vi "ECC_v1.vi"() -> ()   [LabVIEW 2013]
uses:
  state_machine.ctl
  <vilib>/DAQmx/write.llb/DAQmx Write (Analog Wfm 1Chan NSamp).vi
  <vilib>/DAQmx/create/channels.llb/DAQmx Create Channel (AO-Voltage-Basic).vi
  <vilib>/DAQmx/configure/timing.llb/DAQmx Timing (Use Waveform).vi
  <vilib>/DAQmx/miscellaneous.llb/DAQmx Fill In Error Info.vi
panel:
  in  "R&S/5181":bool=TRUE
  out "on_bad_status":bool
  out "off_bad_status":bool
  out "Pause, s":i32
  out "APS_off_status":bool=TRUE
  out "R&S_off_status":bool=TRUE
  out "Countdown":u32
  in  "Rep_delay":u32
  in  "Finite/Continuous":bool
  in  "ResumeSweep":bool
  in  "PauseSweep":bool
  in  "RF_off_rep":bool
  in  "RF_off_set":bool
  in  "RF_off_cycle":bool
  in  "APS_off_rep":bool=TRUE
  in  "APS_off_set":bool
  in  "APS_off_cycle":bool
  in  "AbortSweep":bool
  in  "Check APS":bool
  in  "ON/OFF_APS":bool
  in  "Check R&S":bool
  in  "ON/OFF_RF":bool
  in  "Use_APS":bool=TRUE
  out "DAC_status":bool
  out "RF_status":bool
  out "i_Current_repetition":i32
  out "N_Cycles_Created":i32
  out "i_Current_cycle":i32
  in  "M_repetitions":i32 min=0
  in  "Set_of_Cycles":T1(array[cluster])=[{"On/Off"=TRUE, "f0, MHz"=32.5, "fm, kHz"=100, "A, mV"=20, "Waveform"=enum."triangle", "N_steps"=500, "T_sweep, s"=0.1, "N_sweeps"=5, "End_Wait, s"=0}] {"End_Wait, s" step=1; "N_sweeps" min=0 step=1; "T_sweep, s" min=0.0 step=0.001 format="%#_6f"; "N_steps" min=0 step=1; "fm, kHz" step=1; "f0, MHz" min=0.0 step=0.001 format="%#_6f"}
  out "APS_status":bool
  in  "APS address":refnum<visa-resource-name>="COM3"
  in  "Init Devices":bool
  in  "Do Sweep":bool
  in  "Exit":bool
  in  "DAC channel":tag="Dev1/ao0"
  in  "RF address":string(combo)="29"
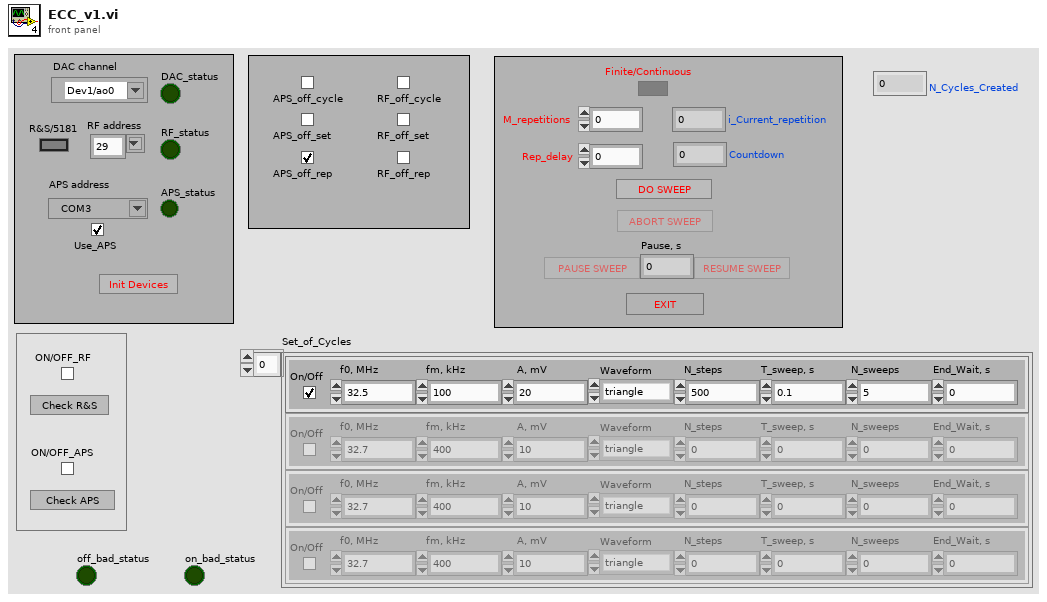
[diagram p1: front panel]
types:
  T1 = cluster{"On/Off":bool, "f0, MHz":dbl, "fm, kHz":i32, "A, mV":i32, "Waveform":enum16{"triangle", "saw_direct", "saw_invert", "sine"}, "N_steps":i32, "T_sweep, s":dbl, "N_sweeps":i32, "End_Wait, s":u32}[]
  T2 = typedef "state_machine.ctl" = enum16{"idle", "init_daq", "init_rf", "init_ps", "cycle_start", "get_wf", "rf_on", "rf_off", "rf_set", "ps_on", "ps_off", "daq_start", "daq_stop", "daq_wait", "daq_dt", "daq_v", "delay", "cycle_reset", "exit", "repetition_reset"}
  T3 = enum8{"Enabled", "Disabled", "Disabled and Grayed Out"}
  T4 = cluster{"On/Off":bool, "f0, MHz":dbl, "fm, kHz":i32, "A, mV":i32, "Waveform":enum16{"triangle", "saw_direct", "saw_invert", "sine"}, "N_steps":i32, "T_sweep, s":dbl, "N_sweeps":i32, "End_Wait, s":u32}
  T5 = enum16{"triangle", "saw_direct", "saw_invert", "sine"}
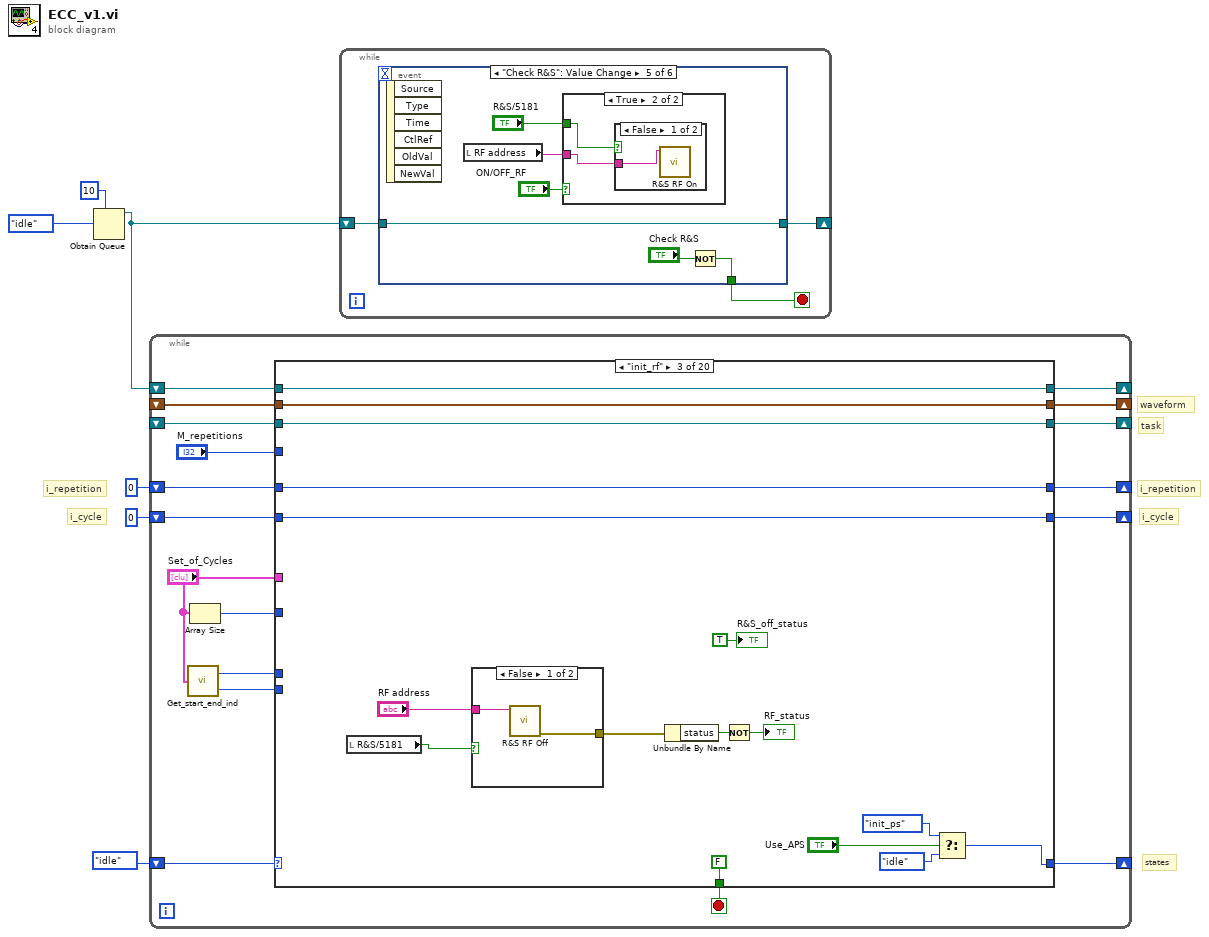
[diagram p0: block diagram]
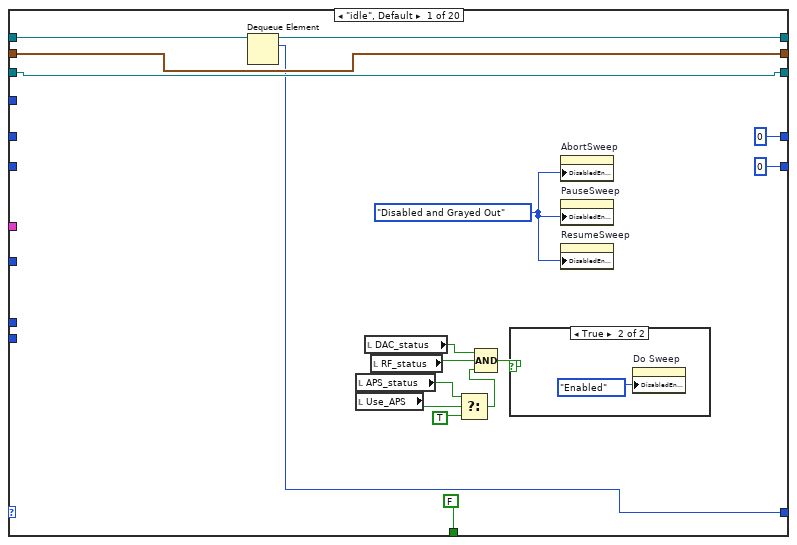
[diagram p2: hidden frame]
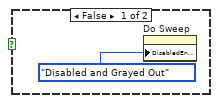
[diagram p3: hidden frame]
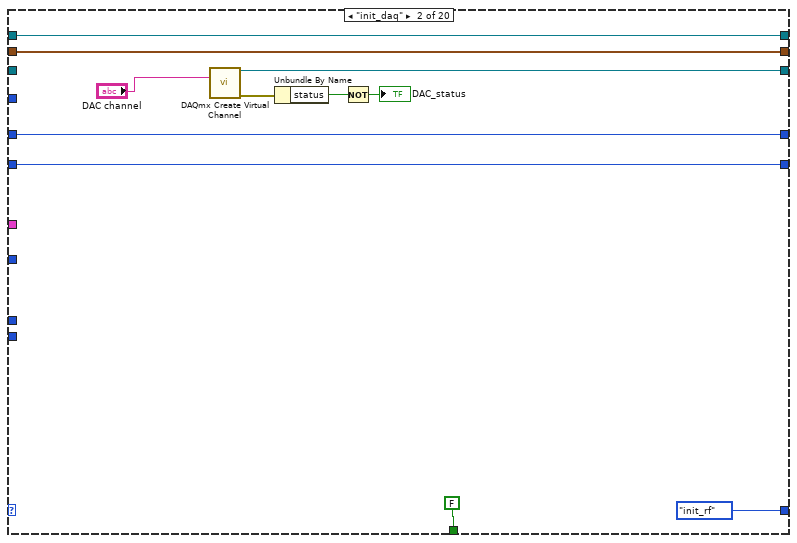
[diagram p4: hidden frame]
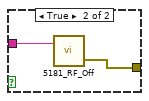
[diagram p5: hidden frame]
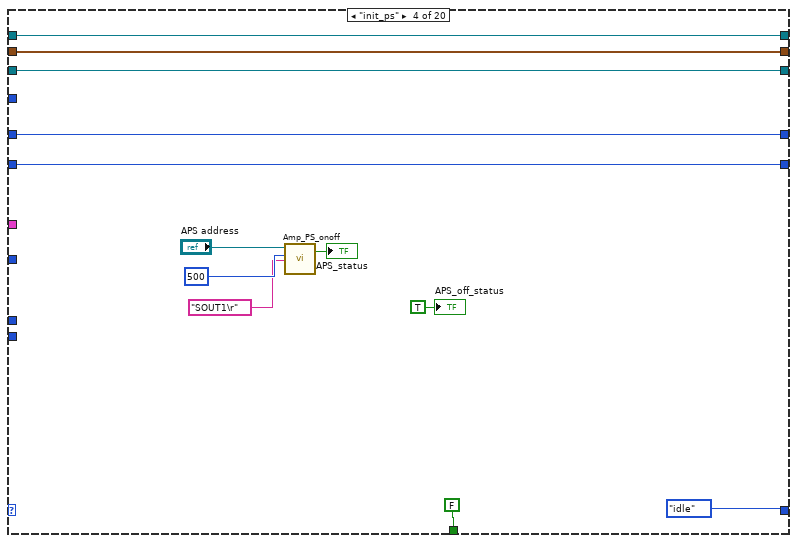
[diagram p6: hidden frame]
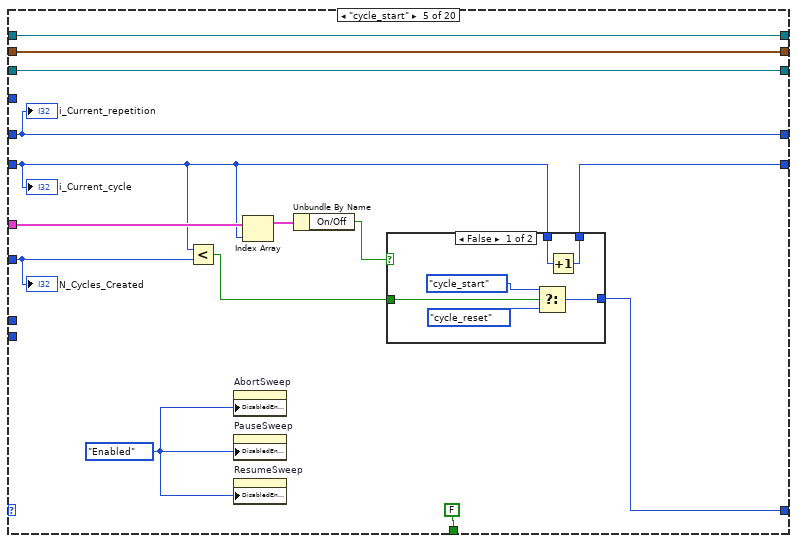
[diagram p7: hidden frame]
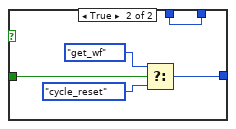
[diagram p8: hidden frame]
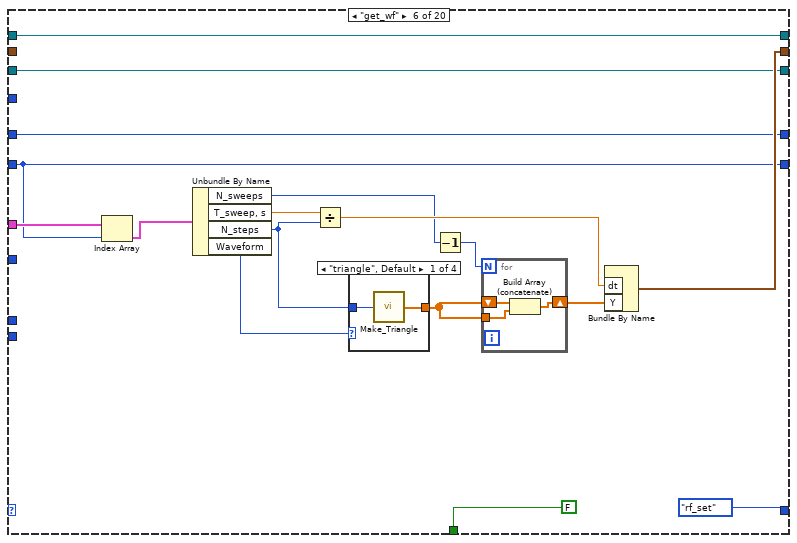
[diagram p9: hidden frame]
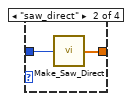
[diagram p10: hidden frame]
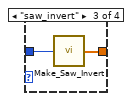
[diagram p11: hidden frame]
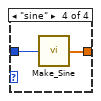
[diagram p12: hidden frame]
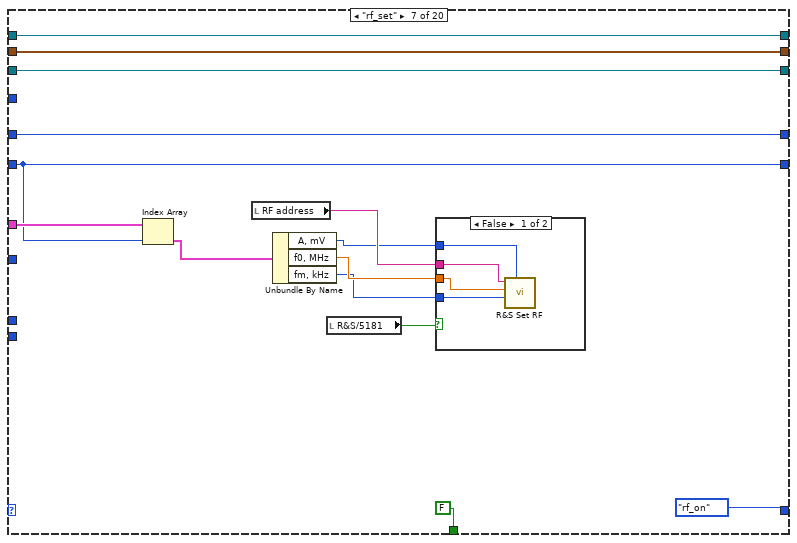
[diagram p13: hidden frame]
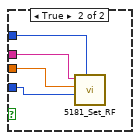
[diagram p14: hidden frame]
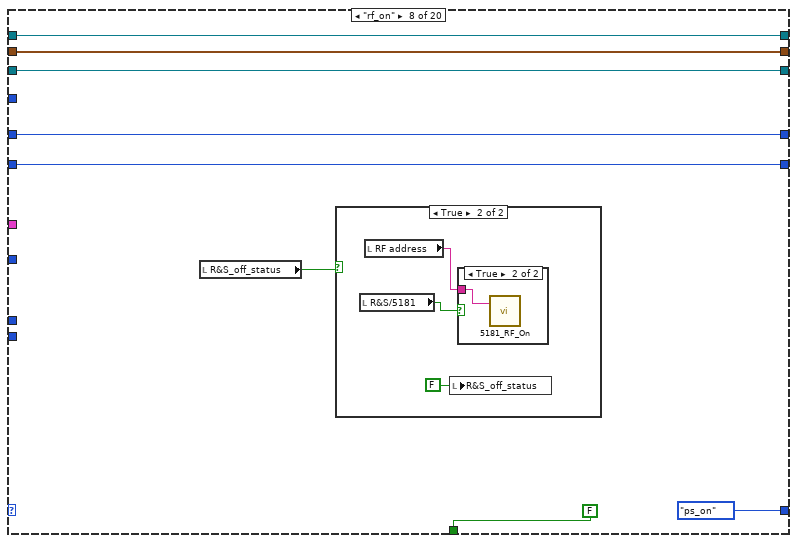
[diagram p15: hidden frame]
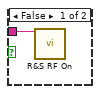
[diagram p17: hidden frame]
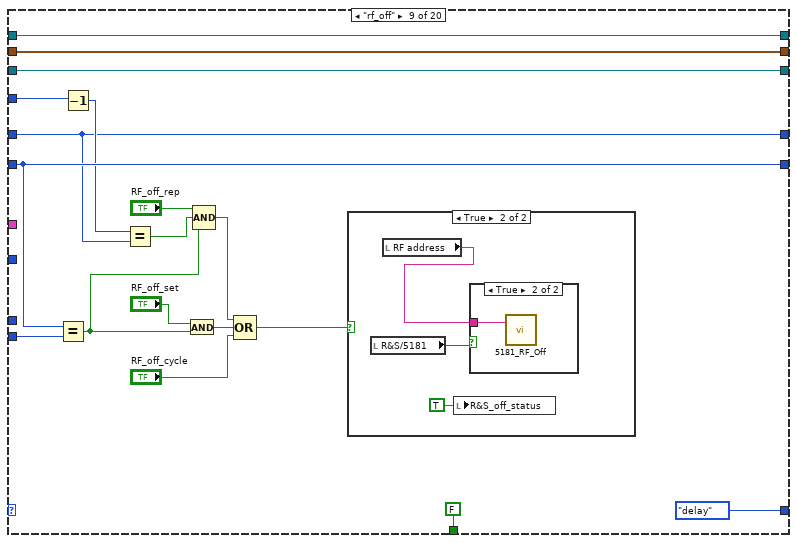
[diagram p18: hidden frame]
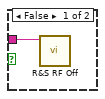
[diagram p20: hidden frame]
diagram:
  # "i_repetition"
  # "i_cycle"
  # "i_repetition"
  # "i_cycle"
  # "states"
  # "waveform"
  # "task"
  n1 = Obtain Queue(max queue size (-1, unlimited)=10, element data type=state_machine."idle") -> (queue out=w4:refnum<queue>)  [unwired: 3 in, 2 out]
  n2 = while {
    shift-right: [w19] -> _
    shift-left: state_machine."idle" -> [w24]
    shift-right: [w23] -> _
    shift-left: _ -> [w21]
    shift-right: [w22] -> _
    shift-left: _ -> [w20]
    shift-right: [w17] -> _
    shift-left: w4 -> [w18]
    shift-right: [w15] -> _
    shift-left: 0 -> [w14]
    shift-right: [w13] -> _
    shift-left: 0 -> [w12]
    stop <- w16 stop-if-true
    n3 = call "Get_start_end_ind.vi"("Set_of_Cycles"="Set_of_Cycles") -> ("start_ind"=w9:i32, "end_ind"=w8:i32)
    n4 = Array Size(array="Set_of_Cycles") -> (size(s)=w11:i32)
    n5 = case shown="\"init_rf\"" w24 {
      selector: w24 -> [_ _ _ _ _ _ _ _ _ _ _ _ _ _ _ _ _ _ w360 _]
      tunnel: [w40 w52 w69 w85 w89 w120 w149 w166 w189 w206 w223 w248 w256 w264 w273 w280 w292 w310 w357 w368] -> w23
      tunnel: "Set_of_Cycles" -> [_ _ _ _ w99 w127 w151 _ _ _ _ _ _ _ _ _ w289 _ _ _]
      tunnel: [w39 w51 w68 w84 w90 w121 w148 w167 w190 w205 w222 w247 w255 w263 w272 w281 w293 w309 w356 w369] -> w22
      tunnel: w21 -> [w40 _ w69 w85 w89 w120 w149 w166 w189 w206 w223 w249 w257 w265 w274 w282 w292 w310 w357 w368]
      tunnel: w20 -> [w39 w51 w68 w84 w90 _ w148 w167 w190 w205 w222 w247 w255 w263 w272 w281 w293 w309 w356 w369]
      tunnel: [w36 state_machine."init_rf" w59 state_machine."idle" w95 state_machine."rf_set" state_machine."rf_on" state_machine."ps_on" state_machine."delay" state_machine."daq_dt" state_machine."rf_off" state_machine."daq_wait" state_machine."ps_off" state_machine."daq_stop" state_machine."daq_v" state_machine."daq_start" state_machine."cycle_start" w308 w360 w364] -> w19
      tunnel: w18 -> [w38 w48 w66 w81 w88 w118 w146 w168 w191 w202 w219 w244 w252 w260 w268 w277 w294 w311 w359 w371]
      tunnel: [w37 w48 w66 w81 w88 w118 w146 w168 w191 w202 w219 w244 w252 w260 w268 w277 w294 w311 w359 w371] -> w17
      tunnel: [FALSE FALSE FALSE FALSE FALSE FALSE FALSE FALSE FALSE FALSE FALSE FALSE FALSE FALSE FALSE FALSE FALSE FALSE TRUE FALSE] -> w16
      tunnel: w11 -> [_ _ _ _ w91 _ _ _ _ _ _ _ _ _ _ _ _ _ _ _]
      tunnel: [0 w47 w65 w80 w94 w111 w144 w162 w185 w200 w217 w243 w251 w259 w267 w276 w284 0 w355 w370] -> w15
      tunnel: w14 -> [_ w47 w65 w80 w92 w111 w144 w162 w185 w200 w217 w243 w251 w259 w267 w276 w283 _ w355 w370]
      tunnel: [0 w46 w64 w79 w87 w113 w145 w165 w177 w201 w212 w242 w250 w258 w266 w275 w291 w305 w354 0] -> w13
      tunnel: w12 -> [_ w46 w64 w79 w87 w113 w145 w165 w177 w201 w212 w242 w250 w258 w266 w275 w291 w306 w354 _]
      tunnel: "M_repetitions" -> [_ _ _ _ _ _ _ _ w182 _ w214 _ _ _ _ _ _ w313 _ _]
      tunnel: w9 -> [_ _ _ _ _ _ _ _ _ _ _ _ _ _ _ _ _ _ _ _]
      tunnel: w8 -> [_ _ _ _ _ _ _ _ w186 _ w218 _ _ _ _ _ _ _ _ _]
      frame "idle", Default {
        w25 = T3."Disabled and Grayed Out" ("Disabled")
        n6 = Dequeue Element(queue=w38) -> (queue out=w37:refnum<queue>, element=w36:T2)  [unwired: 2 in, 2 out]
        n7 = local read "APS_status"() -> (w28:bool)
        n8 = local read "Use_APS"() -> (w30:bool)
        n9 = local read "DAC_status"() -> (w32:bool)
        n10 = local read "RF_status"() -> (w31:bool)
        n11 = Select(t=w28, s=w30, f=TRUE) -> (s? t:f=w27:bool)
        n12 = Compound Arithmetic op=AND(w32, w31, w27) -> (w26:bool)
        n13 = case shown="True" w26 {
          frame False {
            n14 = property on="Do Sweep" class="Bool"("DisabledEnum"=T3."Disabled and Grayed Out" ("Disabled")) -> ()  [unwired: 2 in, 2 out]
          }
          frame True {
            n15 = property on="Do Sweep" class="Bool"("DisabledEnum"=T3."Enabled" ("Disabled")) -> ()  [unwired: 2 in, 2 out]
          }
        }
        n16 = property on="AbortSweep" class="Bool"("DisabledEnum"=w25) -> ()  [unwired: 2 in, 2 out]
        n17 = property on="PauseSweep" class="Bool"("DisabledEnum"=w25) -> ()  [unwired: 2 in, 2 out]
        n18 = property on="ResumeSweep" class="Bool"("DisabledEnum"=w25) -> ()  [unwired: 2 in, 2 out]
      }
      frame "init_daq" {
        n19 = call-poly <vilib>:"DAQmx Create Virtual Channel.vi"("physical channels"="DAC channel") -> ("task out"=w52:refnum<k21>, "error out"=w45:errorcluster)  [unwired: 13 in]
        n20 = Unbundle By Name(w45) -> ("status"=w44:bool)
        n21 = Not(x=w44) -> (.not. x?=→"DAC_status":bool)
      }
      frame "init_rf" {
        n22 = local read "R&S/5181"() -> (w54:bool)
        n23 = case shown="False" w54 {
          tunnel: "RF address" -> [w71 w73]
          tunnel: [w70 w72] -> w55
          frame False {
            n24 = call "R&S RF Off.vi"("address"=w71) -> ("error out"=w70:errorcluster)  [unwired: 5 in, 1 out]
          }
          frame True {
            n25 = call "5181_RF_Off.vi"("address"=w73) -> ("error out"=w72:errorcluster)  [unwired: 1 in, 1 out]
          }
        }
        n26 = Unbundle By Name(w55) -> ("status"=w62:bool)
        n27 = Not(x=w62) -> (.not. x?=→"RF_status":bool)
        n28 = Select(t=state_machine."init_ps", s="Use_APS", f=state_machine."idle") -> (s? t:f=w59:T2)
        "R&S_off_status" <- TRUE ("R&S_off_status")
      }
      frame "init_ps" {
        n29 = call "Amp_PS_onoff.vi"("On/Off Control"="SOUT1\r", "delay before read (ms)"=u32 500, "Amp PS address"="APS address") -> ("status"=→"APS_status":bool)  [unwired: 1 in, 1 out]
        "APS_off_status" <- TRUE ("APS_off_status")
      }
      frame "cycle_start" {
        w86 = T3."Enabled" ("Disabled")
        n30 = Less?(x=w92, y=w91) -> (x < y?=w96:bool)
        n31 = property on="AbortSweep" class="Bool"("DisabledEnum"=w86) -> ()  [unwired: 2 in, 2 out]
        n32 = property on="PauseSweep" class="Bool"("DisabledEnum"=w86) -> ()  [unwired: 2 in, 2 out]
        n33 = property on="ResumeSweep" class="Bool"("DisabledEnum"=w86) -> ()  [unwired: 2 in, 2 out]
        n34 = Index Array(array=w99, index=w92) -> (element=w98:T4)
        n35 = Unbundle By Name(w98) -> ("On/Off"=w97:bool)
        n36 = case shown="False" w97 {
          tunnel: w96 -> [w103 w109]
          tunnel: [w100 w108] -> w95
          tunnel: w92 -> [w105 w106]
          tunnel: [w104 w106] -> w94
          frame False {
            n37 = Select(t=state_machine."cycle_start", s=w103, f=state_machine."cycle_reset") -> (s? t:f=w100:T2)
            n38 = Increment(x=w105) -> (x+1=w104:i32)
          }
          frame True {
            n39 = Select(t=state_machine."get_wf", s=w109, f=state_machine."cycle_reset") -> (s? t:f=w108:T2)
          }
        }
        "N_Cycles_Created" <- w91
        "i_Current_cycle" <- w92
        "i_Current_repetition" <- w87
      }
      frame "get_wf" {
        n40 = Index Array(array=w127, index=w111) -> (element=w126:T4)
        n41 = Unbundle By Name(w126) -> ("N_sweeps"=w117:i32, "T_sweep, s"=w115:dbl, "N_steps"=w114:i32, "Waveform"=w116:T5)
        n42 = Divide(x=w115, y=w114) -> (x/y=w123:dbl)
        n43 = case shown="\"triangle\", Default" w116 {
          tunnel: w114 -> [w132 w134 w136 w138]
          tunnel: [w131 w133 w135 w137] -> w124
          frame "triangle", Default {
            n44 = call "Make_Triangle.vi"("N_steps_1"=w132) -> ("TriangleWaveform"=w131:dbl[])
          }
          frame "saw_direct" {
            n45 = call "Make_Saw_Direct.vi"("N_steps_1"=w134) -> ("SawDirectWaveform"=w133:dbl[])
          }
          frame "saw_invert" {
            n46 = call "Make_Saw_Invert.vi"("N_steps_1"=w136) -> ("SawInvertWaveform"=w135:dbl[])
          }
          frame "sine" {
            n47 = call "Make_Sine.vi"("N_steps_1"=w138) -> ("SineWaveform"=w137:dbl[])
          }
        }
        n48 = Decrement(x=w117) -> (x-1=w122:i32)
        n49 = for {
          N: w122 -> [_]
          shift-right: [w128] -> w125
          shift-left: w124 -> [w130]
          tunnel: w124 -> [w129]
          n50 = Build Array (concatenate)(w130, w129) -> (w128:dbl[])
        }
        n51 = Bundle By Name("dt"=w123, "Y"=w125) -> (w121:waveform(dbl))  [unwired: 1 in]
      }
      frame "rf_set" {
        n52 = Index Array(array=w151, index=w144) -> (element=w150:T4)
        n53 = local read "RF address"() -> (w152:string)
        n54 = Unbundle By Name(w150) -> ("A, mV"=w143:i32, "f0, MHz"=w142:dbl, "fm, kHz"=w141:i32)
        n55 = local read "R&S/5181"() -> (w139:bool)
        n56 = case shown="False" w139 {
          tunnel: w152 -> [w156 w160]
          tunnel: w143 -> [w155 w159]
          tunnel: w142 -> [w154 w158]
          tunnel: w141 -> [w153 w157]
          frame False {
            n57 = call "R&S Set RF.vi"("amplitude (mV)"=w155, "modulation (kHz)"=w153, "center frequency (MHz)"=w154, "address"=w156) -> ()  [unwired: 3 in, 2 out]
          }
          frame True {
            n58 = call "5181_Set_RF.vi"("address"=w160, "center frequency (MHz)"=w158, "modulation (kHz)"=w157, "amplitude (mV)"=w159) -> ()  [unwired: 1 in, 2 out]
          }
        }
      }
      frame "rf_on" {
        n59 = local read "R&S_off_status"() -> (w161:bool)
        n60 = case shown="True" w161 {
          frame False {
          }
          frame True {
            n61 = local read "R&S/5181"() -> (w169:bool)
            n62 = local read "RF address"() -> (w171:string)
            n63 = local write "R&S_off_status"(FALSE ("R&S_off_status")) -> ()
            n64 = case shown="True" w169 {
              tunnel: w171 -> [w172 w173]
              frame False {
                n65 = call "R&S RF On.vi"("address"=w172) -> ()  [unwired: 5 in, 2 out]
              }
              frame True {
                n66 = call "5181_RF_On.vi"("address"=w173) -> ()  [unwired: 1 in, 2 out]
              }
            }
          }
        }
      }
      frame "rf_off" {
        n67 = Equal?(x=w185, y=w186) -> (x = y?=w174:bool)
        n68 = Decrement(x=w182) -> (x-1=w178:i32)
        n69 = Equal?(x=w178, y=w177) -> (x = y?=w175:bool)
        n70 = And(x="RF_off_set", y=w174) -> (x .and. y?=w181:bool)
        n71 = Compound Arithmetic op=AND("RF_off_rep", w175, w174) -> (w179:bool)
        n72 = Compound Arithmetic op=OR(w179, w181, "RF_off_cycle") -> (w183:bool)
        n73 = case shown="True" w183 {
          frame False {
          }
          frame True {
            n74 = local read "R&S/5181"() -> (w192:bool)
            n75 = local read "RF address"() -> (w194:string)
            n76 = local write "R&S_off_status"(TRUE ("R&S_off_status")) -> ()
            n77 = case shown="True" w192 {
              tunnel: w194 -> [w195 w196]
              frame False {
                n78 = call "R&S RF Off.vi"("address"=w195) -> ()  [unwired: 5 in, 2 out]
              }
              frame True {
                n79 = call "5181_RF_Off.vi"("address"=w196) -> ()  [unwired: 1 in, 2 out]
              }
            }
          }
        }
      }
      frame "ps_on" {
        n80 = local read "APS_off_status"() -> (w199:bool)
        n81 = local read "APS_status"() -> (w198:bool)
        n82 = And(x=w198, y=w199) -> (x .and. y?=w197:bool)
        n83 = case shown="True" w197 {
          frame False {
          }
          frame True {
            n84 = local read "APS address"() -> (w209:refnum<visa-resource-name>)
            n85 = local write "APS_off_status"(FALSE ("APS_off_status")) -> ()
            n86 = call "Amp_PS_onoff.vi"("On/Off Control"="SOUT0\r", "delay before read (ms)"=u32 500, "Amp PS address"=w209) -> ("status"=→"on_bad_status":bool)  [unwired: 1 in, 1 out]
          }
        }
      }
      frame "ps_off" {
        n87 = Decrement(x=w214) -> (x-1=w213:i32)
        n88 = local read "APS_status"() -> (w216:bool)
        n89 = case shown="True" w216 {
          selector: w216 -> [w224 _]
          tunnel: w218 -> [_ w236]
          tunnel: w217 -> [_ w235]
          tunnel: [w224 w230] -> w215
          tunnel: w213 -> [_ w226]
          tunnel: w212 -> [_ w227]
          frame False {
          }
          frame True {
            n90 = Equal?(x=w226, y=w227) -> (x = y?=w232:bool)
            n91 = Equal?(x=w235, y=w236) -> (x = y?=w225:bool)
            n92 = Compound Arithmetic op=AND("APS_off_rep", w232, w225) -> (w229:bool)
            n93 = And(x="APS_off_set", y=w225) -> (x .and. y?=w231:bool)
            n94 = Compound Arithmetic op=OR(w229, w231, "APS_off_cycle") -> (w230:bool)
          }
        }
        n95 = case shown="True" w215 {
          frame False {
          }
          frame True {
            n96 = local read "APS address"() -> (w239:refnum<visa-resource-name>)
            n97 = local write "APS_off_status"(TRUE ("APS_off_status")) -> ()
            n98 = call "Amp_PS_onoff.vi"("On/Off Control"="SOUT1\r", "delay before read (ms)"=u32 500, "Amp PS address"=w239) -> ("status"=→"off_bad_status":bool)  [unwired: 1 in, 1 out]
          }
        }
      }
      frame "daq_start" {
        n99 = call <vilib>:"DAQmx Start Task.vi"("task/channels in"=w249) -> ("task out"=w248:refnum<k21>)  [unwired: 13 in, 1 out]
      }
      frame "daq_stop" {
        n100 = call <vilib>:"DAQmx Stop Task.vi"("task/channels in"=w257) -> ("task out"=w256:refnum<k21>)  [unwired: 13 in, 1 out]
      }
      frame "daq_wait" {
        n101 = call <vilib>:"DAQmx Wait Until Done.vi"("task/channels in"=w265) -> ("task out"=w264:refnum<k21>)  [unwired: 13 in, 1 out]
      }
      frame "daq_dt" {
        w271 = 10178 items=["Finite Samples"=10178, "Continuous Samples"=10123, "Hardware Timed Single Point"=12522] ("sample mode")
        n102 = call-poly <vilib>:"DAQmx Timing.vi"("task/channels in"=w274, "sample mode"=w271, "waveform"=w272) -> ("task out"=w273:refnum<k21>)  [unwired: 11 in, 1 out]
      }
      frame "daq_v" {
        n103 = call-poly <vilib>:"DAQmx Write.vi"("task/channels in"=w282, "data"=w281) -> ("task out"=w280:refnum<k21>)  [unwired: 11 in, 2 out]
      }
      frame "delay" {
        # "iterate cycle"
        n104 = Increment(x=w283) -> (x+1=w284:i32)
        n105 = Index Array(array=w289, index=w283) -> (element=w290:T4)
        n106 = Unbundle By Name(w290) -> ("End_Wait, s"=w287:u32)
        n107 = Equal To 0?(x=w287) -> (x = 0?=w288:bool)
        n108 = case shown="True" w288 {
          tunnel: w287 -> [w295 _]
          frame False {
            n109 = Multiply(x=u32 1000 ("y"), y=w295) -> (x*y=w297:u32)
            n110 = Wait (ms)(milliseconds to wait=w297) -> ()  [unwired: 1 out]
          }
          frame True {
          }
        }
      }
      frame "cycle_reset" {
        # "iterate repetition"
        n111 = Increment(x=w306) -> (x+1=w301:i32)
        n112 = case shown="True" "PauseSweep" {
          tunnel: [FALSE ("ResumeSweep") w326] -> w302
          frame False {
          }
          frame True {
            n113 = Tick Count (ms)() -> (millisecond timer value=w327:u32)
            n114 = while {
              tunnel: w327 -> [w333]
              tunnel: ["ResumeSweep"] -> w326
              stop <- "ResumeSweep" stop-if-true
              n115 = Tick Count (ms)() -> (millisecond timer value=w334:u32)
              n116 = Subtract(x=w334, y=w333) -> (x-y=w332:u32)
              n117 = Divide(x=w332, y=u32 1000) -> (x/y=w330:dbl)
              n118 = To Long Integer(number=w330) -> (32bit integer=→"Pause, s":i32)
            }
          }
        }
        n119 = Less?(x=w301, y=w313) -> (x < y?=w307:bool)
        n120 = Or(x="AbortSweep", y="PauseSweep") -> (x .or. y?=w298:bool)
        n121 = case shown="True" "AbortSweep" {
          tunnel: [w343 state_machine."idle"] -> w308
          tunnel: w307 -> [w342 _]
          tunnel: w301 -> [w341 _]
          tunnel: [w341 0] -> w305
          frame False {
            n122 = Select(t=state_machine."cycle_start", s=w342, f=state_machine."repetition_reset") -> (s? t:f=w343:T2)
          }
          frame True {
            w347 = T3."Enabled" ("Disabled")
            n123 = property on="Check APS" class="Bool"("DisabledEnum"=w347) -> ()  [unwired: 2 in, 2 out]
            n124 = property on="Check R&S" class="Bool"("DisabledEnum"=w347) -> ()  [unwired: 2 in, 2 out]
          }
        }
        n125 = case shown="True" w298 {
          frame False {
          }
          frame True {
            n126 = local write "R&S_off_status"(TRUE ("R&S_off_status")) -> ()
            n127 = local read "RF address"() -> (w336:string)
            n128 = call "R&S RF Off.vi"("address"=w336) -> ()  [unwired: 5 in, 2 out]
          }
        }
        n129 = local read "APS_status"() -> (w299:bool)
        n130 = case shown="True" w302 {
          frame False {
          }
          frame True {
            n131 = local read "R&S_off_status"() -> (w320:bool)
            n132 = case shown="False" w320 {
              frame False {
                n133 = local read "RF address"() -> (w324:string)
                n134 = call "R&S RF On.vi"("address"=w324) -> ()  [unwired: 5 in, 2 out]
              }
              frame True {
              }
            }
            n135 = local write "Pause, s"(0 ("Pause, s")) -> ()
            n136 = local read "APS_off_status"() -> (w318:bool)
            n137 = local read "APS_status"() -> (w319:bool)
            n138 = Not(x=w318) -> (.not. x?=w317:bool)
            n139 = And(x=w319, y=w317) -> (x .and. y?=w316:bool)
            n140 = case shown="True" w316 {
              frame False {
              }
              frame True {
                n141 = local read "APS address"() -> (w321:refnum<visa-resource-name>)
                n142 = call "Amp_PS_onoff.vi"("On/Off Control"="SOUT0\r", "delay before read (ms)"=u32 50, "Amp PS address"=w321) -> ()  [unwired: 1 in, 2 out]
              }
            }
          }
        }
        n143 = And(x=w298, y=w299) -> (x .and. y?=w300:bool)
        n144 = case shown="True" w300 {
          frame False {
          }
          frame True {
            n145 = local read "APS address"() -> (w338:refnum<visa-resource-name>)
            n146 = local write "APS_off_status"(TRUE ("APS_off_status")) -> ()
            n147 = call "Amp_PS_onoff.vi"("On/Off Control"="SOUT1\r", "delay before read (ms)"=u32 500, "Amp PS address"=w338) -> ()  [unwired: 1 in, 2 out]
          }
        }
      }
      frame "exit" {
        w349 = FALSE ("DAC_status")
        n148 = local read "APS address"() -> (w352:refnum<visa-resource-name>)
        n149 = local read "Use_APS"() -> (w353:bool)
        n150 = local read "RF address"() -> (w351:string)
        n151 = case shown="False" w353 {
          tunnel: w352 -> [_ w361]
          frame False {
          }
          frame True {
            n152 = call "Amp_PS_onoff.vi"("On/Off Control"="SOUT1\r", "delay before read (ms)"=u32 50, "Amp PS address"=w361) -> ()  [unwired: 1 in, 2 out]
          }
        }
        n153 = call "R&S RF Off.vi"("address"=w351) -> ()  [unwired: 5 in, 2 out]
        n154 = property on="Init Devices" class="Bool"("DisabledEnum"=T3."Enabled" ("Disabled")) -> ()  [unwired: 2 in, 2 out]
        n155 = local write "DAC_status"(w349) -> ()
        n156 = local write "RF_status"(w349) -> ()
        n157 = local write "APS_status"(w349) -> ()
      }
      frame "repetition_reset" {
        n158 = case shown="True" "Finite/Continuous" {
          tunnel: [state_machine."idle" state_machine."cycle_start"] -> w364
          frame False {
          }
          frame True {
            n159 = Tick Count (ms)() -> (millisecond timer value=w374:u32)
            n160 = while {
              tunnel: w374 -> [w381]
              tunnel: "Rep_delay" -> [w377]
              stop <- w379 stop-if-true
              w376 = u32 1000 ("y")
              n161 = Tick Count (ms)() -> (millisecond timer value=w382:u32)
              n162 = Subtract(x=w382, y=w381) -> (x-y=w383:u32)
              n163 = Divide(x=w383, y=w376) -> (x/y=w384:dbl)
              n164 = Wait (ms)(milliseconds to wait=w376) -> ()  [unwired: 1 out]
              n165 = To Long Integer(number=w384) -> (32bit integer=w378:i32)
              n166 = Subtract(x=w377, y=w378) -> (x-y=w380:u32)
              "Countdown" <- w380
              n167 = Less Or Equal To 0?(x=w380) -> (x <= 0?=w379:bool)
            }
          }
        }
      }
    }
  }
  n168 = while {
    shift-right: [w385] -> _
    shift-left: w4 -> [w386]
    stop <- w387 stop-if-true
    n169 = event shown="[4] \"Check R&S\": Value Change" {
      selector: _ -> [_ _ _ _ _ _]
      dyn-events: _ -> [_ _ _ _ _ _]
      timeout: _ -> [_ _ _ _ _ _]
      tunnel: [_ "Exit" w397 w403 w410 w423] -> w387
      tunnel: w386 -> [w388 w391 w396 w402 w407 w420]
      tunnel: [w388 w390 w395 w401 w407 w420] -> w385
      event Timeout {
        n170 = event-data() -> ()  [unwired: 1 in, 3 out]
      }
      event "Exit": Value Change {
        n171 = event-data() -> ()  [unwired: 1 in, 6 out]
        n172 = Enqueue Element(queue=w391, element=state_machine."exit") -> (queue out=w390:refnum<queue>)  [unwired: 2 in, 2 out]
      }
      event "Init Devices": Value Change {
        n173 = event-data() -> ()  [unwired: 1 in, 6 out]
        n174 = Enqueue Element(queue=w396, element=state_machine."init_daq") -> (queue out=w395:refnum<queue>)  [unwired: 2 in, 2 out]
        n175 = property on="Init Devices" class="Bool"("DisabledEnum"=T3."Disabled and Grayed Out" ("Disabled")) -> ()  [unwired: 2 in, 2 out]
        n176 = Not(x="Init Devices") -> (.not. x?=w397:bool)
      }
      event "Do Sweep": Value Change {
        w399 = T3."Disabled and Grayed Out" ("Disabled")
        n177 = event-data() -> ()  [unwired: 1 in, 6 out]
        n178 = Enqueue Element(queue=w402, element=state_machine."cycle_start") -> (queue out=w401:refnum<queue>)  [unwired: 2 in, 2 out]
        n179 = Not(x="Do Sweep") -> (.not. x?=w403:bool)
        n180 = property on="Check R&S" class="Bool"("DisabledEnum"=w399) -> ()  [unwired: 2 in, 2 out]
        n181 = property on="Check APS" class="Bool"("DisabledEnum"=w399) -> ()  [unwired: 2 in, 2 out]
      }
      event "Check R&S": Value Change {
        n182 = event-data() -> ()  [unwired: 1 in, 6 out]
        n183 = local read "RF address"() -> (w408:string)
        n184 = case shown="True" "ON/OFF_RF" {
          tunnel: w408 -> [w412 w416]
          tunnel: "R&S/5181" -> [w411 w415]
          frame False {
            n185 = case shown="True" w411 {
              tunnel: w412 -> [w413 w414]
              frame False {
                n186 = call "R&S RF Off.vi"("address"=w413) -> ()  [unwired: 5 in, 2 out]
              }
              frame True {
                n187 = call "5181_RF_Off.vi"("address"=w414) -> ()  [unwired: 1 in, 2 out]
              }
            }
          }
          frame True {
            n188 = case shown="False" w415 {
              tunnel: w416 -> [w417 w418]
              frame False {
                n189 = call "R&S RF On.vi"("address"=w417) -> ()  [unwired: 5 in, 2 out]
              }
              frame True {
                n190 = call "5181_RF_On.vi"("address"=w418) -> ()  [unwired: 1 in, 2 out]
              }
            }
          }
        }
        n191 = Not(x="Check R&S") -> (.not. x?=w410:bool)
      }
      event "Check APS": Value Change {
        n192 = event-data() -> ()  [unwired: 1 in, 6 out]
        n193 = local read "APS address"() -> (w421:refnum<visa-resource-name>)
        n194 = case shown="False" "ON/OFF_APS" {
          tunnel: w421 -> [w424 w427]
          frame False {
            n195 = call "Amp_PS_onoff.vi"("On/Off Control"="SOUT1\r", "delay before read (ms)"=u32 50, "Amp PS address"=w424) -> ()  [unwired: 1 in, 2 out]
          }
          frame True {
            n196 = call "Amp_PS_onoff.vi"("On/Off Control"="SOUT0\r", "delay before read (ms)"=u32 50, "Amp PS address"=w427) -> ()  [unwired: 1 in, 2 out]
          }
        }
        n197 = Not(x="Check APS") -> (.not. x?=w423:bool)
      }
    }
  }
